vi "Configure Reference Oscillator.vi"(8 "error in (no error)":errorcluster, 10 "Reference Mode":enum16{"Internal", "External"}(ring), 11 "PSG-MXG in":refnum<class "PSG-MXG.lvclass">) -> (0 "error out":errorcluster, 3 "PSG-MXG out":refnum<class "PSG-MXG.lvclass">)   [LabVIEW 2020, in "PSG-MXG.lvclass"]
uses:
  PSG-MXG.lvclass
  C:/Sandbox/RF Bench/Source Code/WiSpry Test Framework/Instruments/Instrument.lvclass
  C:/Sandbox/RF Bench/Source Code/WiSpry Test Framework/Instruments/Signal Generator/Signal Generator.lvclass
  Instrument.lvclass/Instrument.ctl
  Signal Generator.lvclass/Signal Generator.ctl
  Instrument.lvclass
  Signal Generator.lvclass
  <instrlib>/Agilent PSG MXG Series/Agilent PSG MXG Series.lvlib
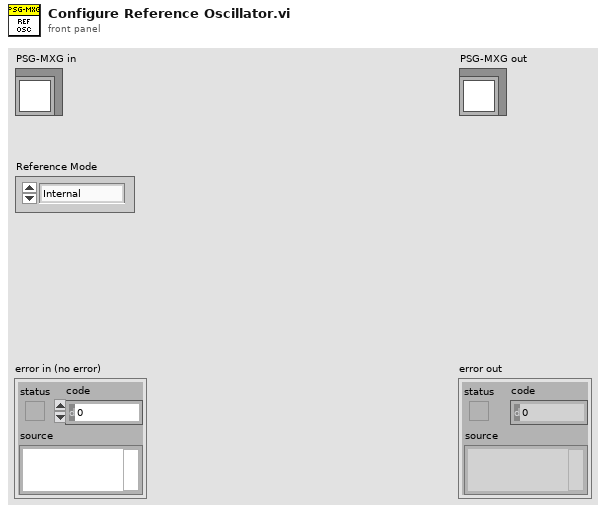
[diagram p1: front panel]
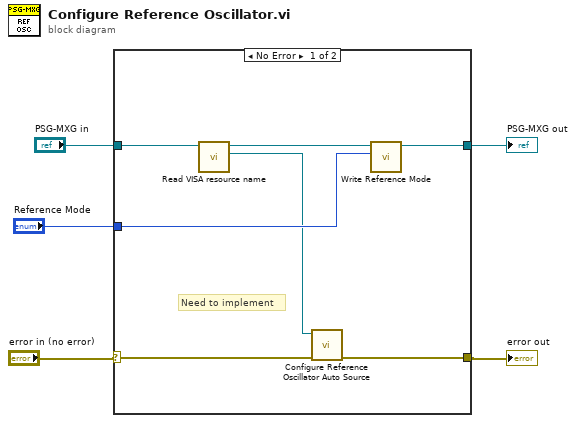
[diagram p0: block diagram]
diagram:
  n1 = case shown="No Error" "error in (no error)" {
    selector: "error in (no error)" -> [w8 w14]
    tunnel: "PSG-MXG in" -> [w12 w13]
    tunnel: [w7 w14] -> w4
    tunnel: [w10 w13] -> w3
    tunnel: "Reference Mode" -> [w9 _]
    frame No Error {
      # "Need to implement"
      n2 = call "Read VISA resource name.vi"("Instrument in"=w12) -> ("VISA resource name"=w6:refnum<visa-resource-name>, "Instrument out"=w11:refnum<class "PSG-MXG.lvclass">)  [unwired: 9 in]
      n3 = call <instrlib>:"Configure Reference Oscillator Auto Source.vi"("error in (no error)"=w8, "VISA resource name"=w6) -> ("error out"=w7:errorcluster)  [unwired: 8 in, 1 out]
      n4 = call "Write Reference Mode.vi"("Reference Mode"=w9, "Signal Generator in"=w11) -> ("Signal Generator out"=w10:refnum<class "PSG-MXG.lvclass">)  [unwired: 9 in]
    }
    frame Error {
    }
  }
  "error out" <- w4
  "PSG-MXG out" <- w3
